vi "Get Initial Colors.vi"(8 "error in (no error)":errorcluster, 11 "senseHatDisplay in":refnum<class "RPI.SenseHat.Display.lvclass">) -> (0 "error out":errorcluster, 2 "Initial Colors":refnum<class "Color.lvclass">[][](array[class]), 3 "senseHatDisplay out":refnum<class "RPI.SenseHat.Display.lvclass">)   [LabVIEW 2020, in "RPI.SenseHat.Display.lvlib" / "RPI.SenseHat.Display.lvclass"]
doc: "Returns the start-up rainbow colors."
uses:
  RPI.SenseHat.Display.lvclass
  Color/Color.lvclass
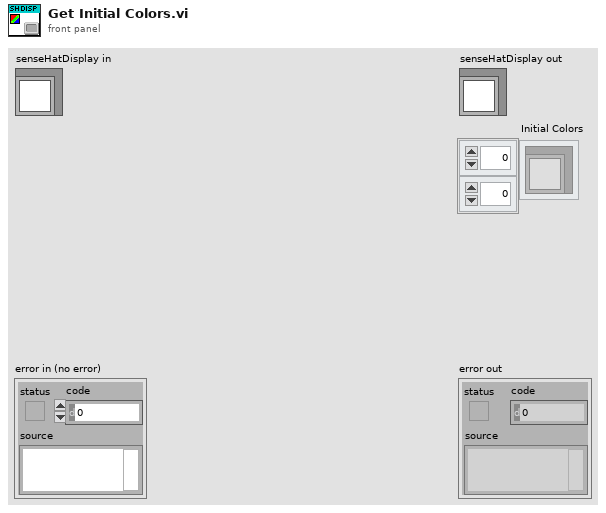
[diagram p1: front panel]
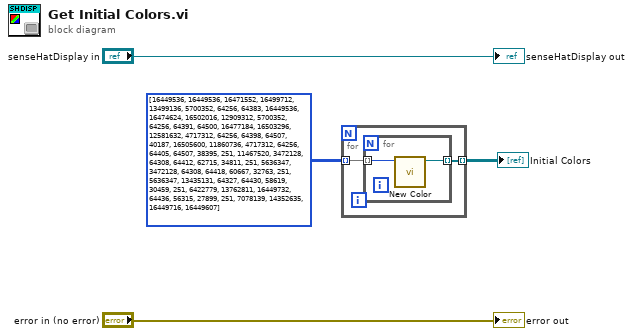
[diagram p0: block diagram]
diagram:
  n1 = for {
    tunnel: u32[][] [[16449536, 16449536, 16471552, 16499712, 13499136, 5700352, 64256, 64383], [16449536, 16474624, 16502016, 12909312, 5700352, 64256, 64391, 64500], [16477184, 16503296, 12581632, 4717312, 64256, 64398, 64507, 40187], [16505600, 11860736, 4717312, 64256, 64405, 64507, 38395, 251], [11467520, 3472128, 64308, 64412, 62715, 34811, 251, 5636347], [3472128, 64308, 64418, 60667, 32763, 251, 5636347, 13435131], [64327, 64430, 58619, 30459, 251, 6422779, 13762811, 16449732], [64436, 56315, 27899, 251, 7078139, 14352635, 16449716, 16449607]] ("Initial Colors") -> [w6] mode=indexing
    tunnel: [w5] -> w1 mode=indexing
    n2 = for {
      tunnel: w6 -> [w8] mode=indexing
      tunnel: [w7] -> w5 mode=indexing
      n3 = call "New Color.vi"("Color Box"=w8) -> ("Color out"=w7:refnum<class "Color.lvclass">)  [unwired: 9 in, 1 out]
    }
  }
  "Initial Colors" <- w1
  "error out" <- "error in (no error)"
  "senseHatDisplay out" <- "senseHatDisplay in"
